vi "Get Point Cloud Data.vi"(8 "error in (no error)":errorcluster, 11 "LiDAR in":refnum<class "LiDAR.lvclass">) -> (0 "error out":errorcluster, 3 "LiDAR out":refnum<class "LiDAR.lvclass">)   [LabVIEW 2018, in "LiDAR.lvlib" / "LiDAR.lvclass"]
uses:
  LiDAR.lvclass
  Controls/cls_Point_Cloud_Packet_Header.ctl
  Controls/cls_Point_Cloud_Return_Data.ctl
panel:
  out "Pount Cloud Data out":T1
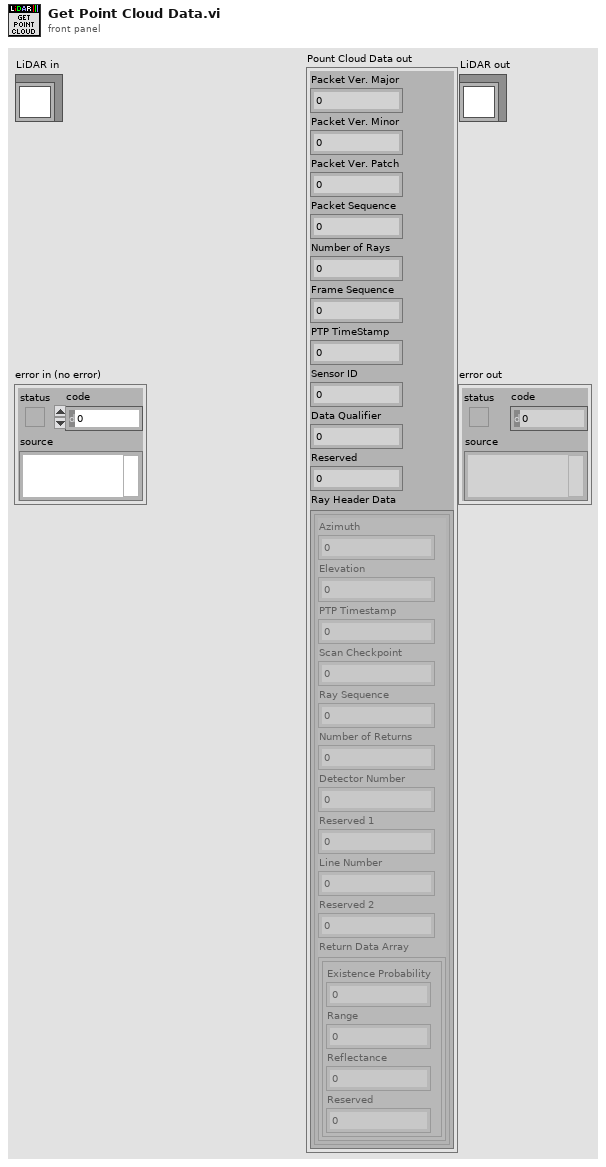
[diagram p1: front panel]
types:
  T1 = typedef "LiDAR.lvlib/LiDAR.lvclass/cls_Point_Cloud_Packet_Header.ctl" = cluster{"Packet Ver. Major":u8, "Packet Ver. Minor":u8, "Packet Ver. Patch":u8, "Packet Sequence":u8, "Number of Rays":u8, "Frame Sequence":u8, "PTP TimeStamp":u64, "Sensor ID":u8, "Data Qualifier":u8, "Reserved":u16, "Ray Header Data":cluster{"Azimuth":u16, "Elevation":u16, "PTP Timestamp":u32, "Scan Checkpoint":u8, "Ray Sequence":u8, "Number of Returns":u8, "Detector Number":u8, "Reserved 1":u8, "Line Number":u16, "Reserved 2":u32, "Return Data Array":T2[]}[]}
  T2 = typedef "LiDAR.lvlib/LiDAR.lvclass/cls_Point_Cloud_Return_Data.ctl" = cluster{"Existence Probability":u8, "Range":u32, "Reflectance":u16, "Reserved":u16}
  T3 = typedef "LiDAR.lvlib/LiDAR.lvclass/cls_Point_Cloud_Ray_Header.ctl" = cluster{"Azimuth":u16, "Elevation":u16, "PTP Timestamp":u32, "Scan Checkpoint":u8, "Ray Sequence":u8, "Number of Returns":u8, "Detector Number":u8, "Reserved 1":u8, "Line Number":u16, "Reserved 2":u32, "Return Data Array":T2[]}
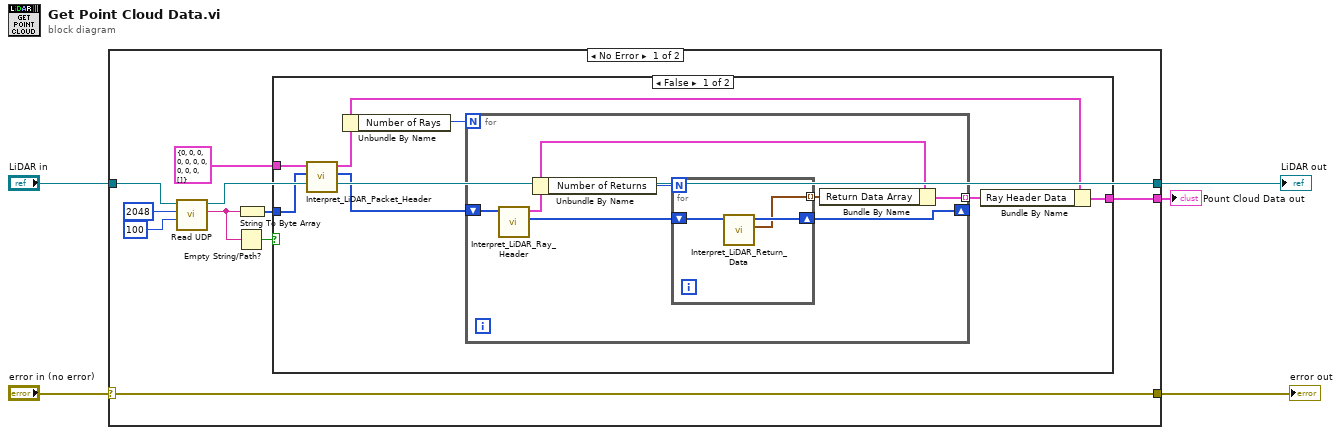
[diagram p0: block diagram]
diagram:
  n1 = case shown="No Error" "error in (no error)" {
    selector: "error in (no error)" -> [w15 w34]
    tunnel: [w15 w34] -> w4
    tunnel: [w8 w33] -> w2
    tunnel: "LiDAR in" -> [w9 w33]
    tunnel: [w7 _] -> w1
    frame No Error {
      n2 = call-dynamic "Read UDP.vi"("Timeout (ms)"=100, "Max Size"=2048, "LiDAR in"=w9) -> ("String"=w11:string, "LiDAR out"=w8:refnum<class "LiDAR.lvclass">)  [unwired: 6 in, 1 out]
      n3 = Empty String/Path?(string/path=w11) -> (empty?=w12:bool)
      n4 = String To Byte Array(string=w11) -> (unsigned byte array=w10:u8[])
      n5 = case shown="False" w12 {
        tunnel: T1 {"Packet Ver. Major"=0, "Packet Ver. Minor"=0, "Packet Ver. Patch"=0, "Packet Sequence"=0, "Number of Rays"=0, "Frame Sequence"=0, "PTP TimeStamp"=0, "Sensor ID"=0, "Data Qualifier"=0, "Reserved"=0, "Ray Header Data"=[]} ("Point Cloud LiDAR Packet Header") -> [w22 _]
        tunnel: w10 -> [w21 _]
        tunnel: [w16 _] -> w7
        frame False {
          n6 = call "Interpret_LiDAR_Packet_Header.vi"("Data in"=w21, "Point Cloud LiDAR Packet Header"=w22) -> ("Remaining Data out"=w20:u8[], "output cluster"=w18:T1)  [unwired: 8 in]
          n7 = Unbundle By Name(w18) -> ("Number of Rays"=w19:u8)
          n8 = for {
            N: w19 -> [_]
            shift-right: [w24] -> _
            shift-left: w20 -> [w29]
            tunnel: [w23] -> w17 mode=indexing
            n9 = call "Interpret_LiDAR_Ray_Header.vi"("Data in"=w29) -> ("Remaining Data out"=w27:u8[], "output cluster"=w26:T3)  [unwired: 9 in]
            n10 = Unbundle By Name(w26) -> ("Number of Returns"=w28:u8)
            n11 = for {
              N: w28 -> [_]
              shift-right: [w31] -> w24
              shift-left: w27 -> [w32]
              tunnel: [w30] -> w25 mode=indexing
              n12 = call "Interpret_LiDAR_Return_Data.vi"("Remaining Data in"=w32) -> ("Return Data out"=w30:T2, "Remaining Data out"=w31:u8[])  [unwired: 9 in]
            }
            n13 = Bundle By Name(cluster=w26, "Return Data Array"=w25) -> (w23:T3)
          }
          n14 = Bundle By Name(cluster=w18, "Ray Header Data"=w17) -> (w16:T1)
        }
        frame True {
        }
      }
    }
    frame Error {
    }
  }
  "error out" <- w4
  "LiDAR out" <- w2
  "Pount Cloud Data out" <- w1
